vi "PartAddLine(SubVI).vi"(8 "error in (no error)":errorcluster, 9 "element in":T1 {"Color" format="%x"}, 10 "String in":string, 11 "ComboBox in":refnum<vi>) -> (0 "error out":errorcluster, 3 "element out":T1 {"Color" format="%x"})   [LabVIEW 2018]
uses:
  CTL/Line.ctl
  Windows/Settings/View.ctl
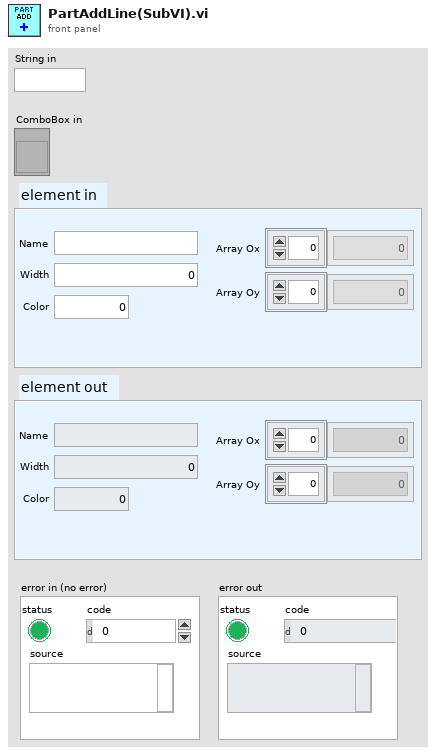
[diagram p1: front panel]
types:
  T1 = typedef "Line.ctl" = cluster{"Width":dbl, "Color":i64, "Array Oy":dbl[], "Array Ox":dbl[], "Name":string, "Plot Visible":T2}
  T2 = typedef "View.ctl" = bool
  T3 = typedef "LVComboBoxStrsAndValuesArrayTypeDef.ctl" = cluster{"String":string, "Value":string}[]
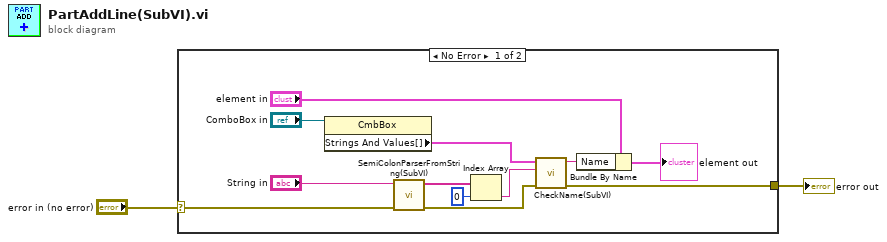
[diagram p0: block diagram]
diagram:
  n1 = case shown="No Error" "error in (no error)" {
    selector: "error in (no error)" -> [w6 w15]
    tunnel: [w4 w15] -> w1
    frame No Error {
      n2 = property on="Property Node" class="CmbBox"(reference="ComboBox in") -> ("Strings And Values[]"=w11:T3)  [unwired: 1 in, 2 out]
      n3 = call "SemiColonParserFromString(SubVI).vi"("Error In"=w6, "String In"="String in") -> ("Error Out"=w5:errorcluster, "String Array Out"=w9:string[])  [unwired: 8 in]
      n4 = Index Array(array=w9, index=0) -> (element=w7:string)
      n5 = call "CheckName(SubVI).vi"("Error In"=w5, "Name In"=w7, "Strings And Values[]"=w11) -> ("Error Out"=w4:errorcluster, "Name Out"=w10:string)  [unwired: 7 in]
      n6 = Bundle By Name(cluster="element in", "Name"=w10) -> (→"element out":T1)
    }
    frame Error {
    }
  }
  "error out" <- w1
